vi "parameters table ROI - inverse.vi"(8 "error in":errorcluster, 10 "Edit Cluster":T1, 11 "data ROIs In":T2) -> (0 "error out":errorcluster, 3 "data ROIs Out":T2)   [LabVIEW 2023]
uses:
  control/rois list cluster.ctl
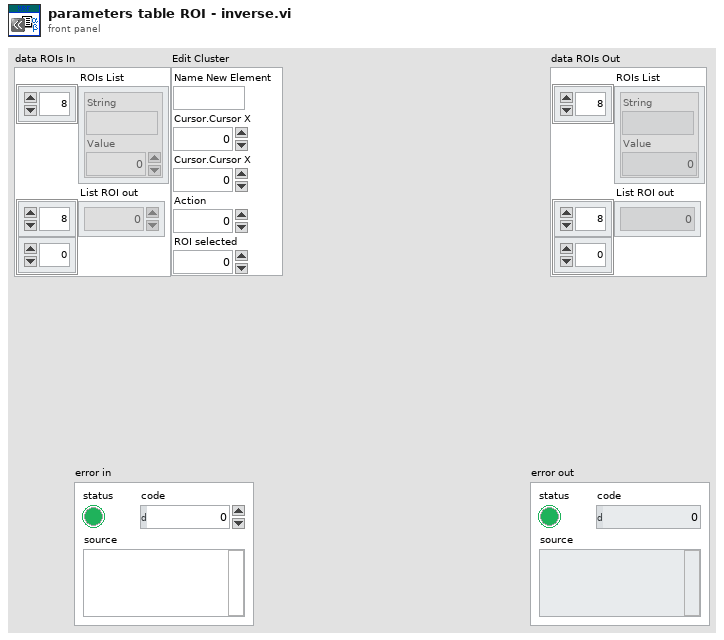
[diagram p1: front panel]
types:
  T1 = cluster{"Name New Element":string, "Cursor.Cursor X":dbl, "Cursor.Cursor X":dbl, "Action":u16, "ROI selected":i16}
  T2 = typedef "rois list cluster.ctl" = cluster{"ROIs List":cluster{"String":string, "Value":i32}[], "List ROI out":dbl[][]}
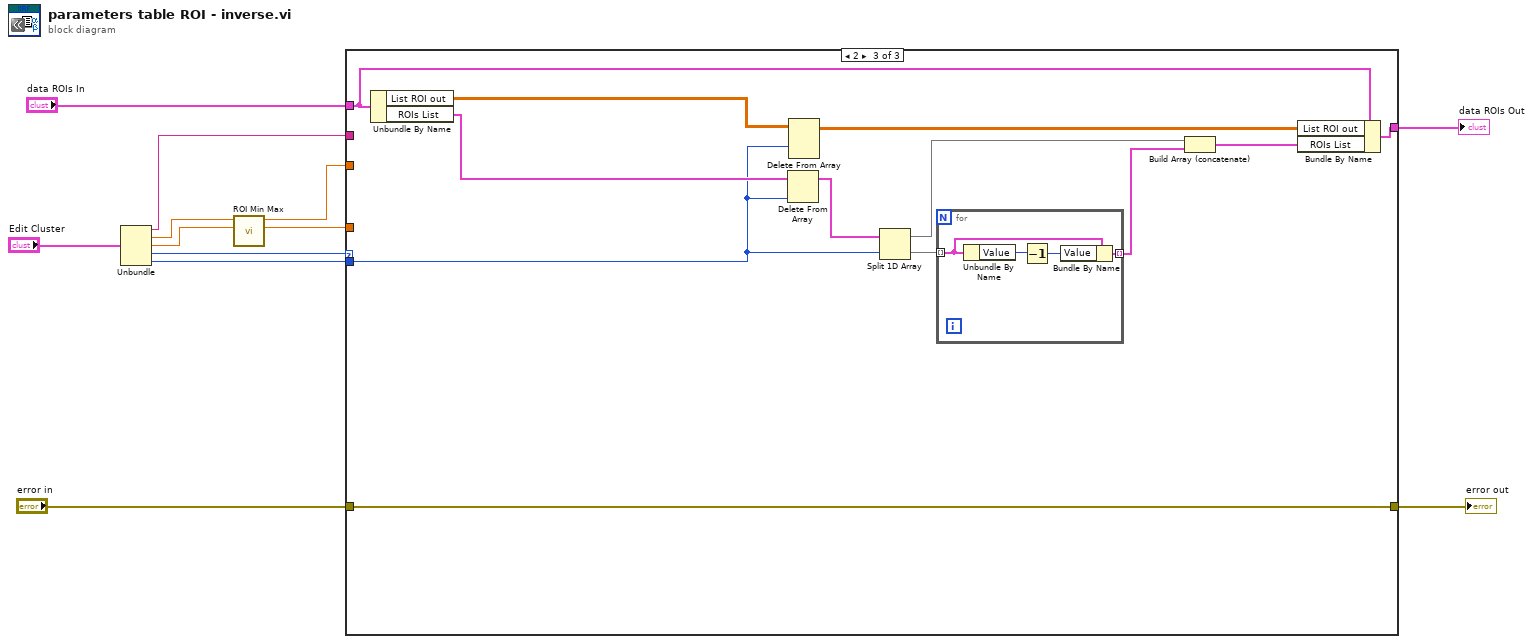
[diagram p0: block diagram]
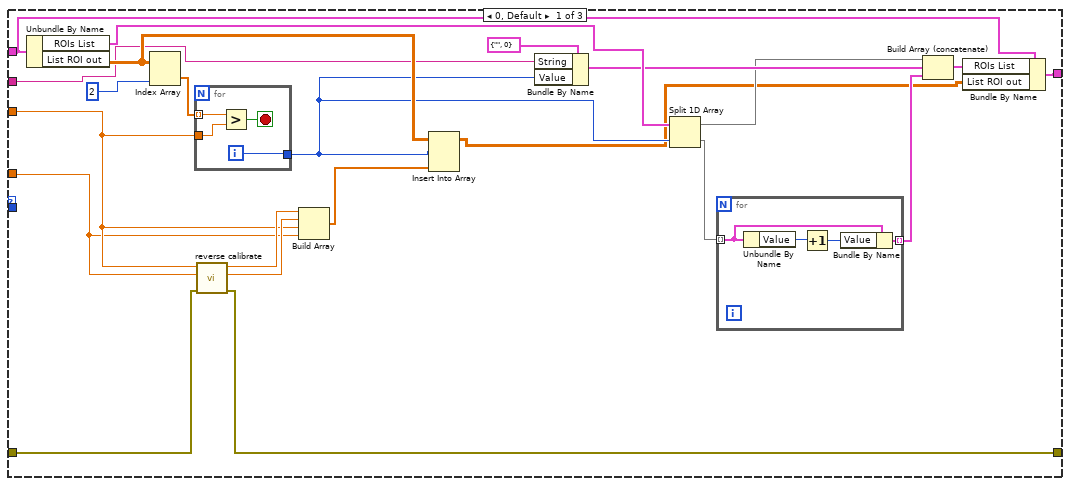
[diagram p2: hidden frame]
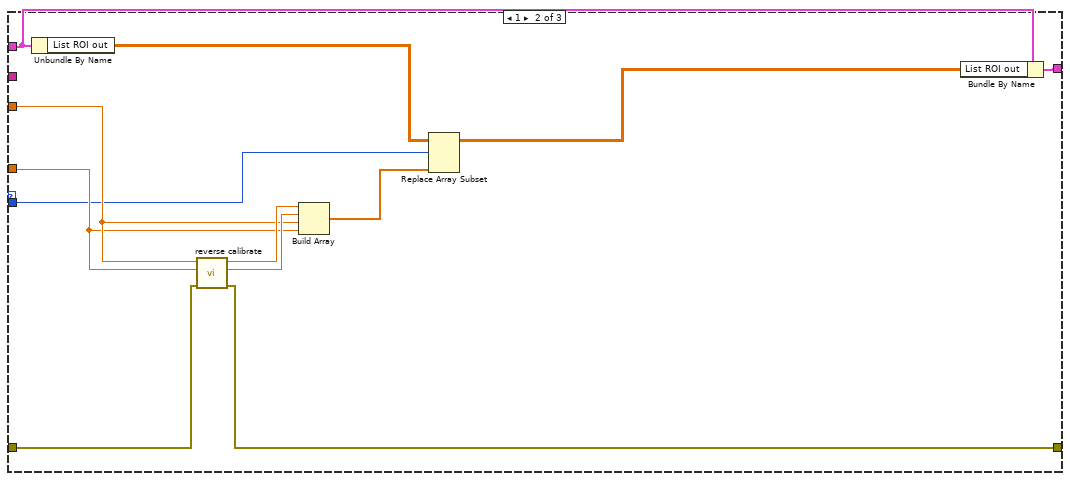
[diagram p3: hidden frame]
diagram:
  n1 = Unbundle("Edit Cluster") -> ("Name New Element"=w7:string, "Cursor.Cursor X"=w4:dbl, "Cursor.Cursor X"=w3:dbl, "Action"=w11:u16, "ROI selected"=w8:i16)
  n2 = call "ROI Min Max.vi"("ROI 2"=w3, "ROI 1"=w4) -> ("ROI Max"=w1:dbl, "ROI Min"=w2:dbl)  [unwired: 8 in]
  n3 = case shown="2" w11 {
    tunnel: "error in" -> [w14 w48 w64]
    tunnel: "data ROIs In" -> [w18 w50 w66]
    tunnel: w2 -> [w30 w52 _]
    tunnel: w1 -> [w29 w51 _]
    tunnel: w8 -> [_ w43 w59]
    tunnel: w7 -> [w25 _ _]
    tunnel: [w15 w49 w65] -> w6
    tunnel: [w13 w47 w64] -> w5
    frame 0, Default {
      n4 = Unbundle By Name(w18) -> ("ROIs List"=w24:cluster{"String":string, "Value":i32}[], "List ROI out"=w27:dbl[][])
      n5 = Index Array(array=w27, index (col)=2 ("index (row)")) -> (element=w34:dbl[])  [unwired: 1 in]
      n6 = for {
        tunnel: w34 -> [w42] mode=indexing
        tunnel: w30 -> [w41]
        tunnel: [w39] -> w23
        i -> [w39]
        stop <- w40 stop-if-true
        n7 = Greater?(x=w42, y=w41) -> (0:w40:bool)
      }
      n8 = call "reverse calibrate.vi"("error in"=w14, "Energy Max"=w29, "Energy Min"=w30) -> ("error out"=w13:errorcluster, "Channel Max"=w31:dbl, "Channel Min"=w32:dbl)  [unwired: 6 in]
      n9 = Build Array(w32, w31, w30, w29) -> (w28:dbl[])
      n10 = Insert Into Array(array=w27, index (row)=w23, new element=w28) -> (w16:dbl[][])  [unwired: 1 in]
      n11 = Bundle By Name(cluster=cluster{"String":string, "Value":i16} {"String"="", "Value"=0}, "String"=w25, "Value"=w23) -> (w20:cluster{"String":string, "Value":i16})
      n12 = Split 1D Array(array=w24, index=w23) -> (first subarray=w19:cluster{"String":string, "Value":i32}[], second subarray=w22:cluster{"String":string, "Value":i32}[])
      n13 = for {
        tunnel: w22 -> [w36] mode=indexing
        tunnel: [w35] -> w21 mode=indexing
        n14 = Unbundle By Name(w36) -> ("Value"=w38:i32)
        n15 = Increment(x=w38) -> (x+1=w37:i32)
        n16 = Bundle By Name(cluster=w36, "Value"=w37) -> (w35:cluster{"String":string, "Value":i32})
      }
      n17 = Build Array (concatenate)(w19, w20, w21) -> (w17:cluster{"String":string, "Value":i32}[])
      n18 = Bundle By Name(cluster=w18, "ROIs List"=w17, "List ROI out"=w16) -> (w15:T2)
    }
    frame 1 {
      n19 = Unbundle By Name(w50) -> ("List ROI out"=w46:dbl[][])
      n20 = call "reverse calibrate.vi"("error in"=w48, "Energy Max"=w51, "Energy Min"=w52) -> ("error out"=w47:errorcluster, "Channel Max"=w53:dbl, "Channel Min"=w54:dbl)  [unwired: 6 in]
      n21 = Build Array(w54, w53, w52, w51) -> (w45:dbl[])
      n22 = Replace Array Subset(array=w46, new element=w45, index (row)=w43) -> (w44:dbl[][])  [unwired: 1 in]
      n23 = Bundle By Name(cluster=w50, "List ROI out"=w44) -> (w49:T2)
    }
    frame 2 {
      n24 = Unbundle By Name(w66) -> ("List ROI out"=w63:dbl[][], "ROIs List"=w61:cluster{"String":string, "Value":i32}[])
      n25 = Delete From Array(array=w61, index=w59) -> (array with subset deleted=w58:cluster{"String":string, "Value":i32}[])  [unwired: 1 in, 1 out]
      n26 = Delete From Array(array=w63, index (row)=w59) -> (array with subset deleted=w62:dbl[][])  [unwired: 2 in, 1 out]
      n27 = Split 1D Array(array=w58, index=w59) -> (first subarray=w55:cluster{"String":string, "Value":i32}[], second subarray=w60:cluster{"String":string, "Value":i32}[])
      n28 = for {
        tunnel: w60 -> [w68] mode=indexing
        tunnel: [w67] -> w57 mode=indexing
        n29 = Unbundle By Name(w68) -> ("Value"=w70:i32)
        n30 = Decrement(x=w70) -> (x-1=w69:i32)
        n31 = Bundle By Name(cluster=w68, "Value"=w69) -> (w67:cluster{"String":string, "Value":i32})
      }
      n32 = Build Array (concatenate)(w55, w57) -> (w56:cluster{"String":string, "Value":i32}[])
      n33 = Bundle By Name(cluster=w66, "List ROI out"=w62, "ROIs List"=w56) -> (w65:T2)
    }
  }
  "error out" <- w5
  "data ROIs Out" <- w6
